vi "login.vi"() -> ()   [LabVIEW 2017]
panel:
  out "bandera 2":bool
  out "Usuarios dados de alta":string[][](array[string])
  out "Control":enum32{"LOGIN", "MENU 1", "MENU 2"}(tab)
  in  "ingresar  2":bool
  in  "Contraseña 2":string
  in  "Usuario 2":string
  in  "volver 3":bool
  in  "Agragar usuario 2":bool
  in  "Usuario  2":string
  in  "Contraseña 3":string
  out "Secion iniciada por: 2":string
  in  "eliminar 2":bool
  in  "Digite el usuario que desea eliminar 2":string
  in  "OK Button 2":bool
  in  "volver 4":bool
  out "bandera":bool
  out "Usuarios dados de alta":string[][](array[string])
  out "Control":enum32{"LOGIN", "MENU 1", "MENU 2"}(tab)
  in  "ingresar":bool
  in  "Contraseña":string
  in  "Usuario":string
  in  "volver":bool
  in  "Agragar usuario":bool
  in  "Usuario":string
  in  "Contraseña":string
  out "Secion iniciada por:":string
  in  "eliminar":bool
  in  "Digite el usuario que desea eliminar":string
  in  "OK Button":bool
  in  "volver 2":bool
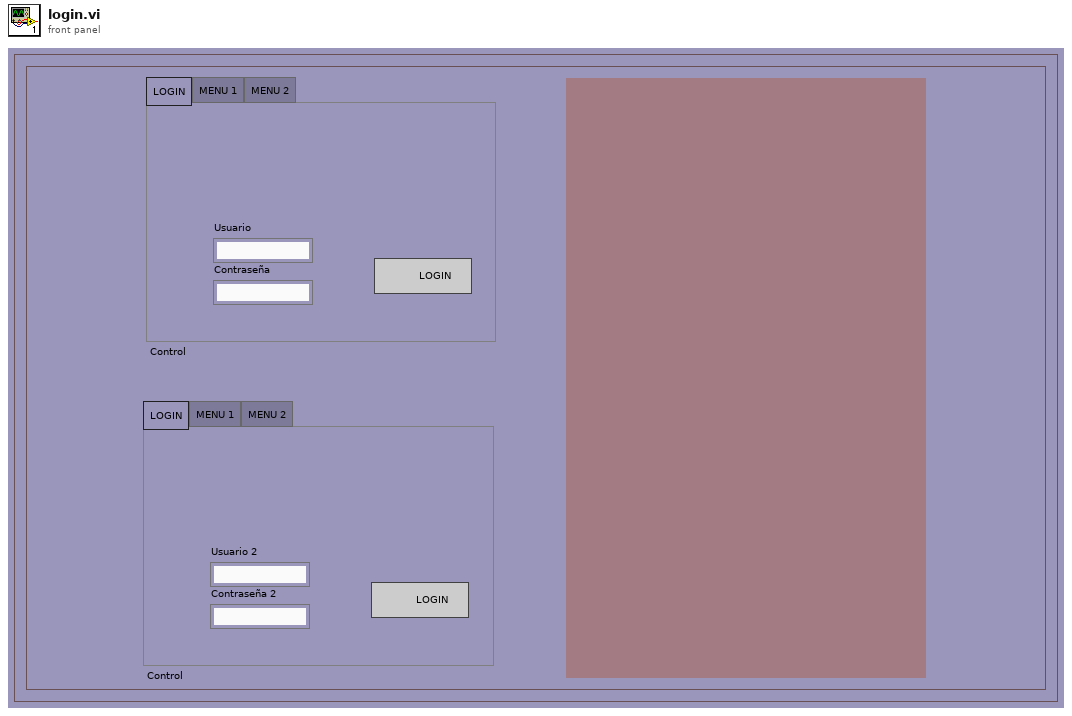
[diagram p1: front panel]
types:
  T1 = enum16{"open", "replace", "create", "open or create", "replace or create", "replace or create with confirmation"}
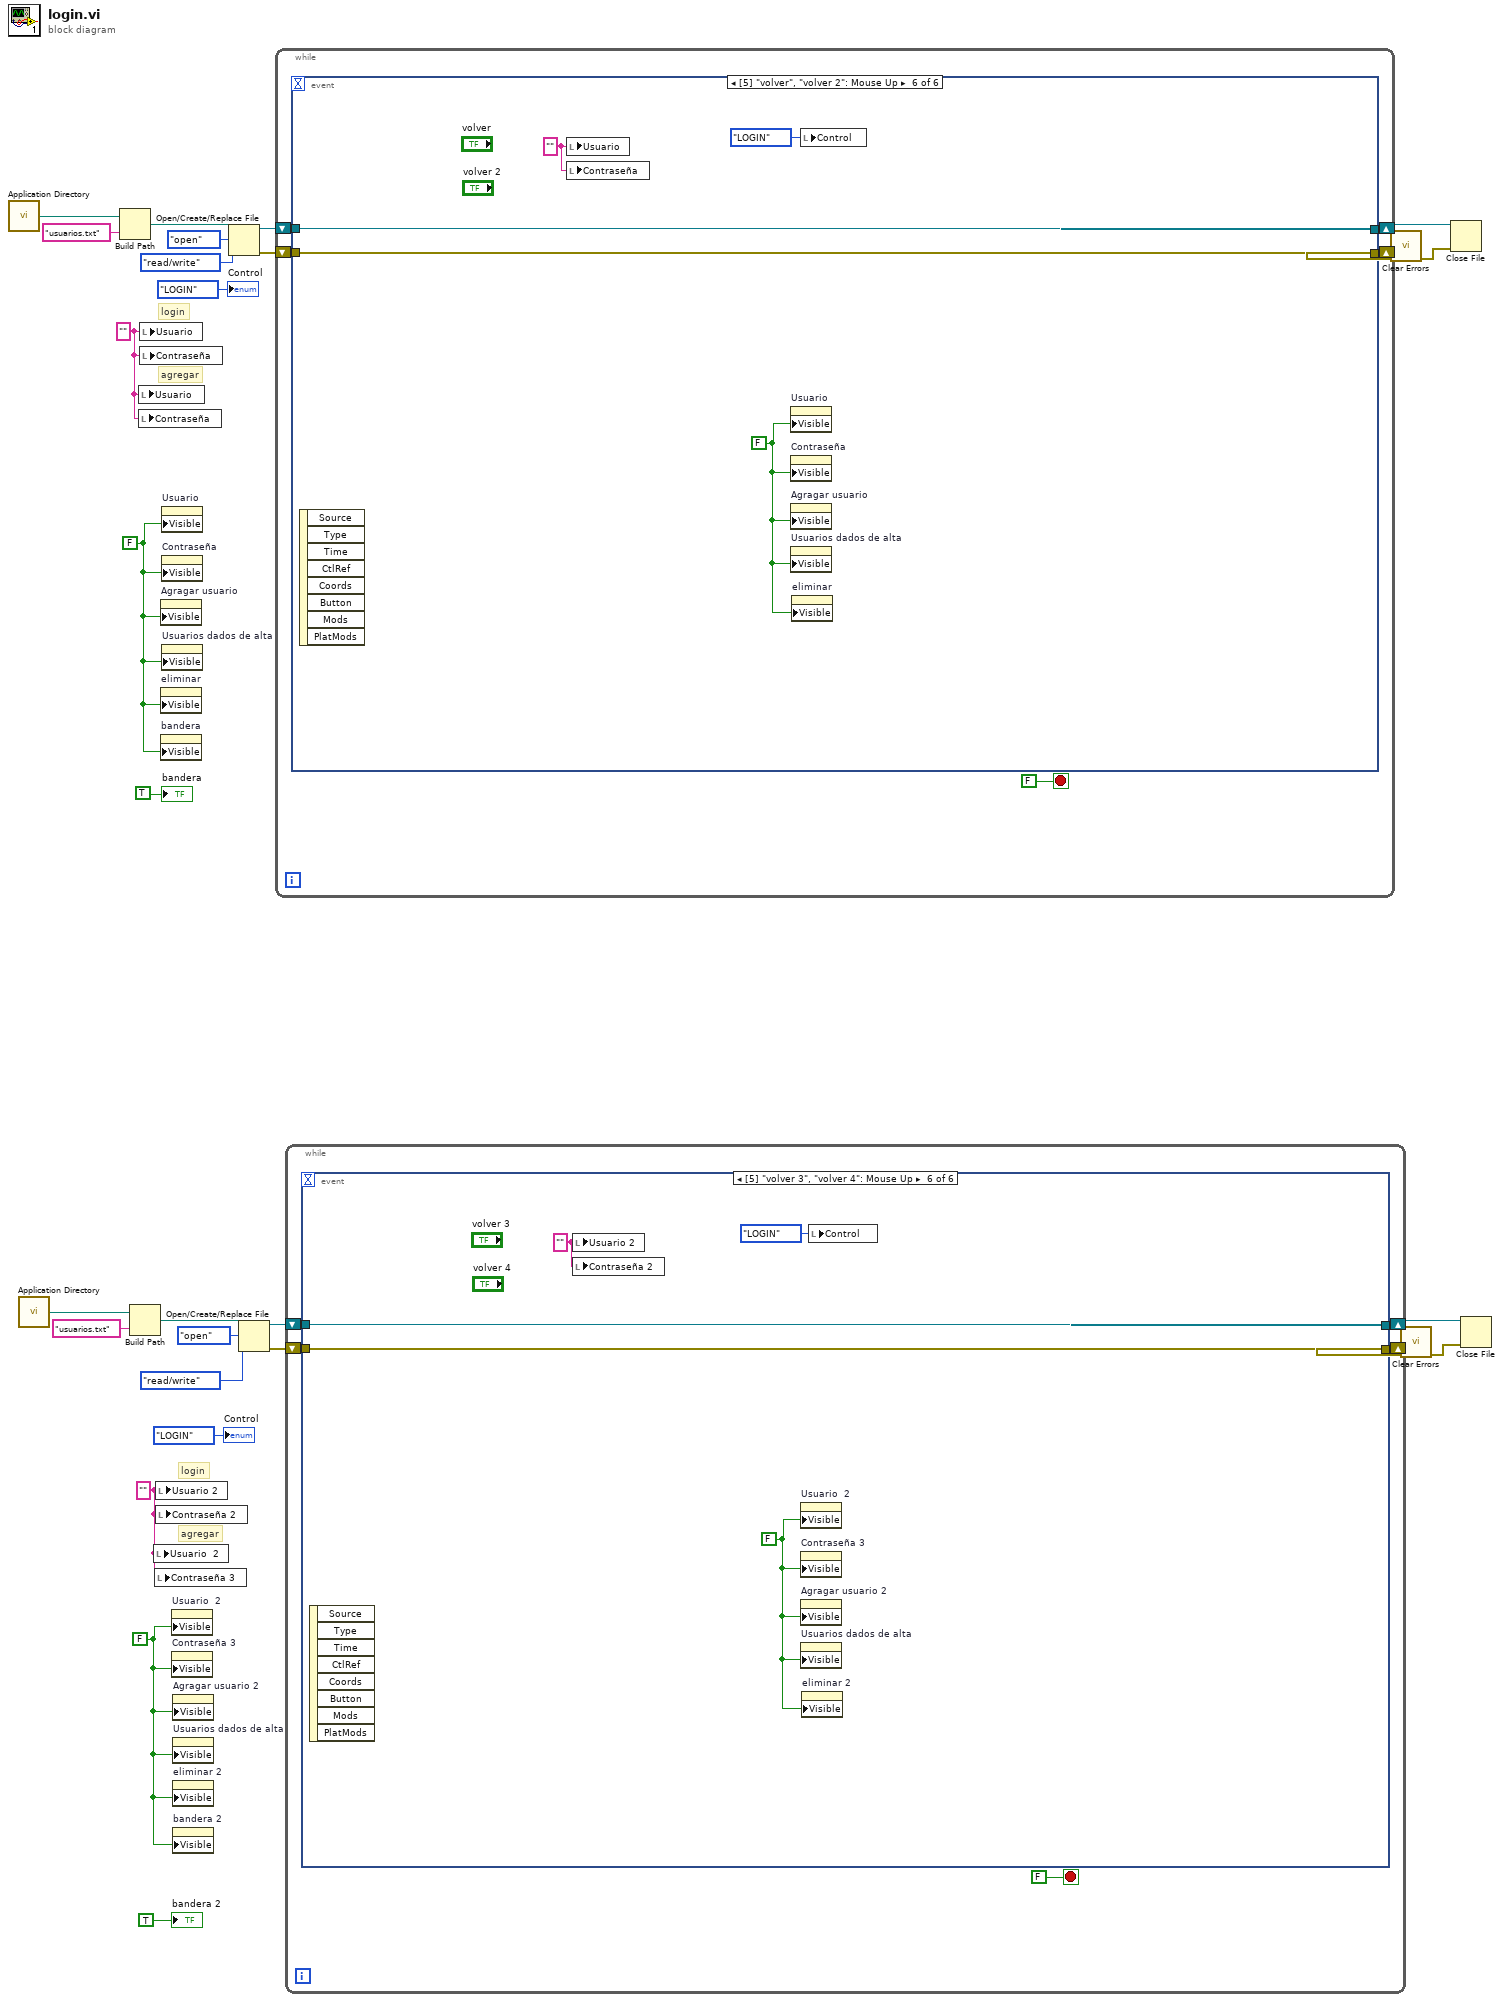
[diagram p0: block diagram]
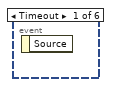
[diagram p2: hidden frame]
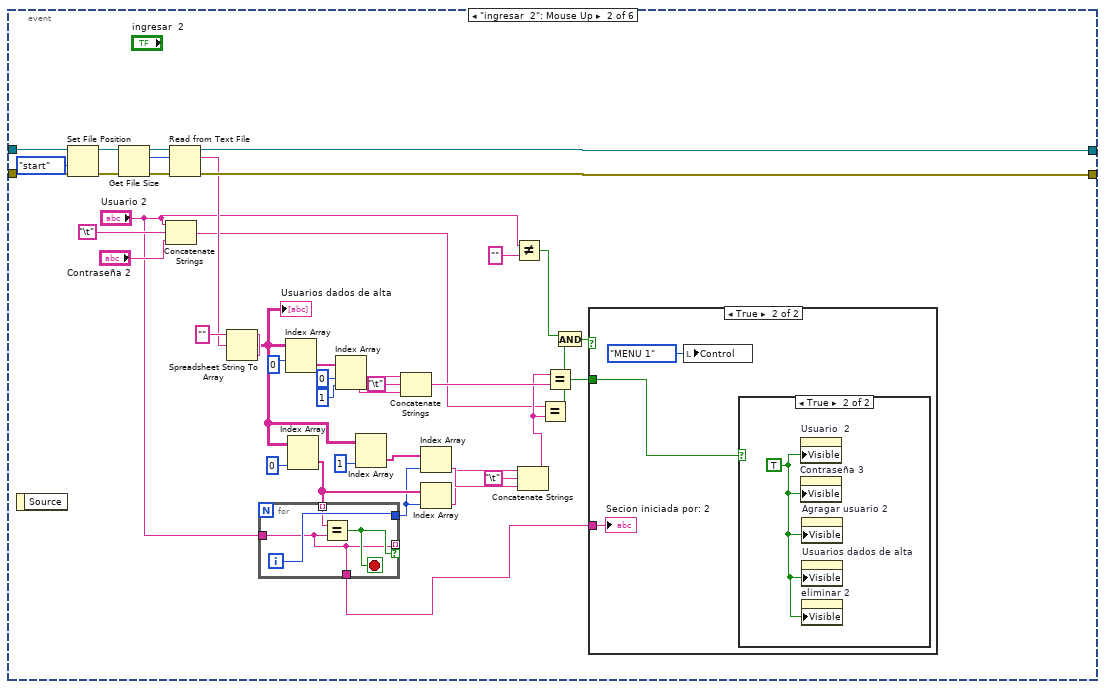
[diagram p3: hidden frame]
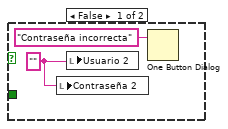
[diagram p4: hidden frame]
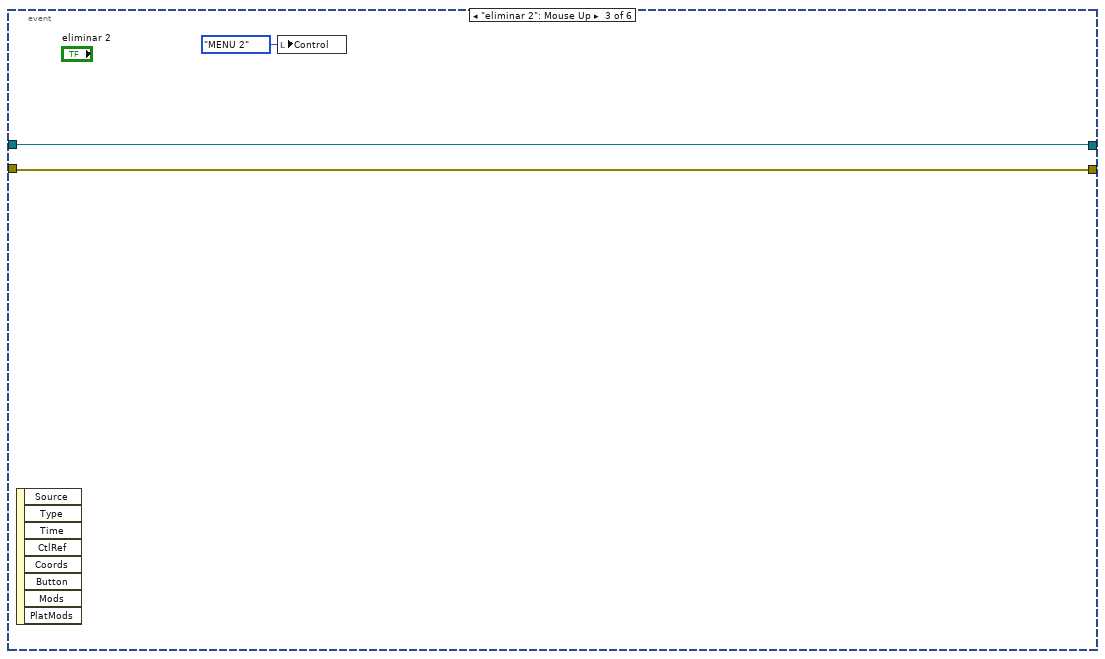
[diagram p6: hidden frame]
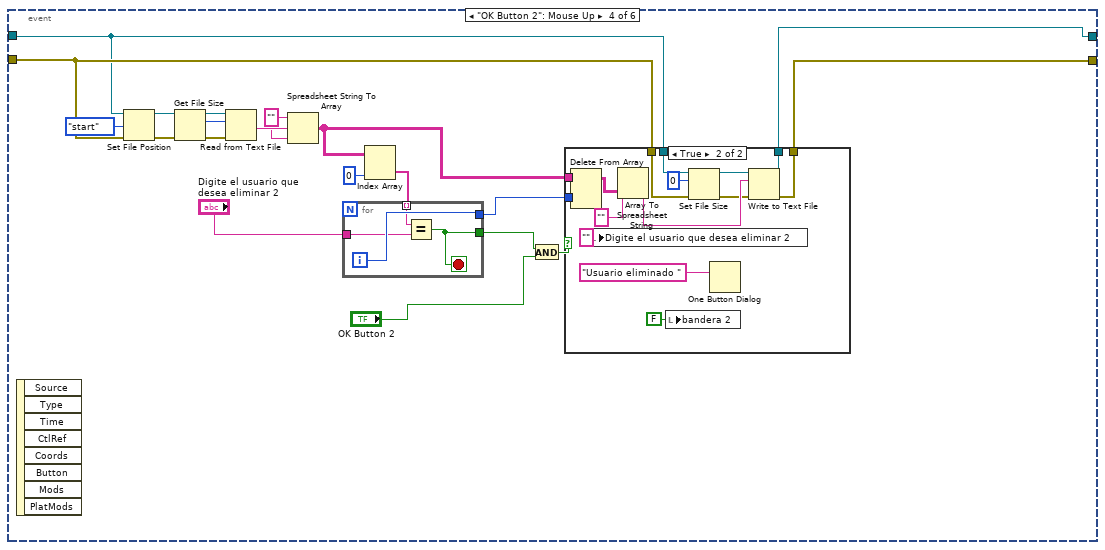
[diagram p7: hidden frame]
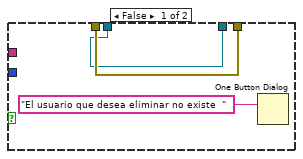
[diagram p8: hidden frame]
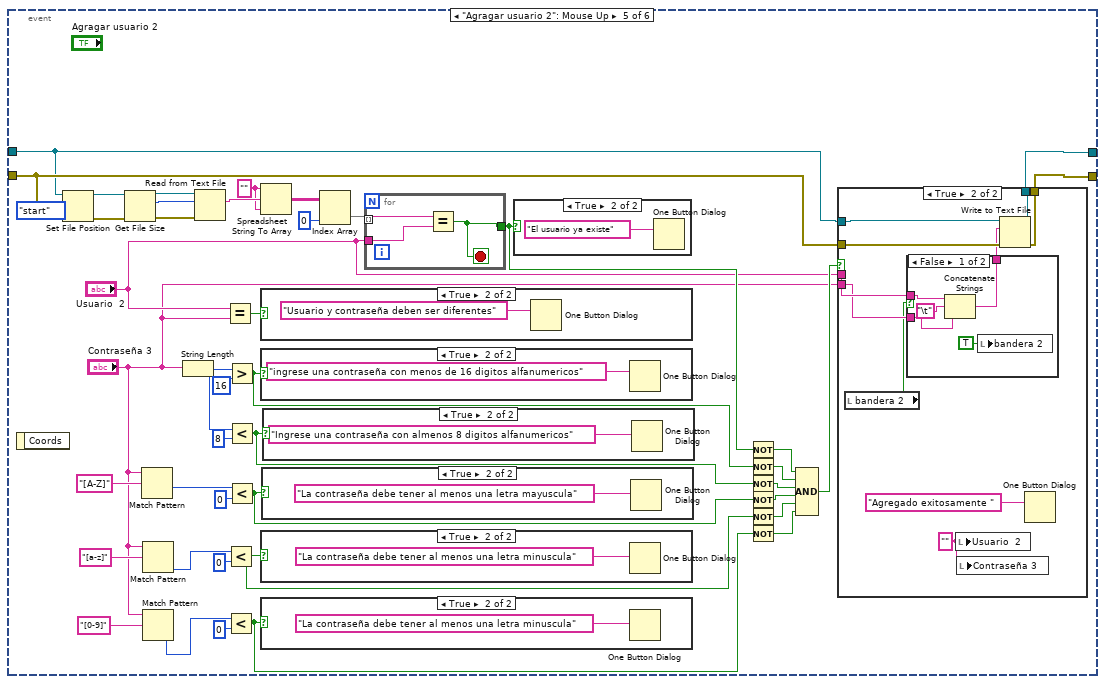
[diagram p9: hidden frame]
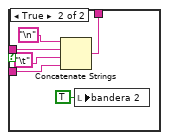
[diagram p11: hidden frame]
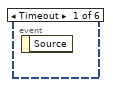
[diagram p19: hidden frame]
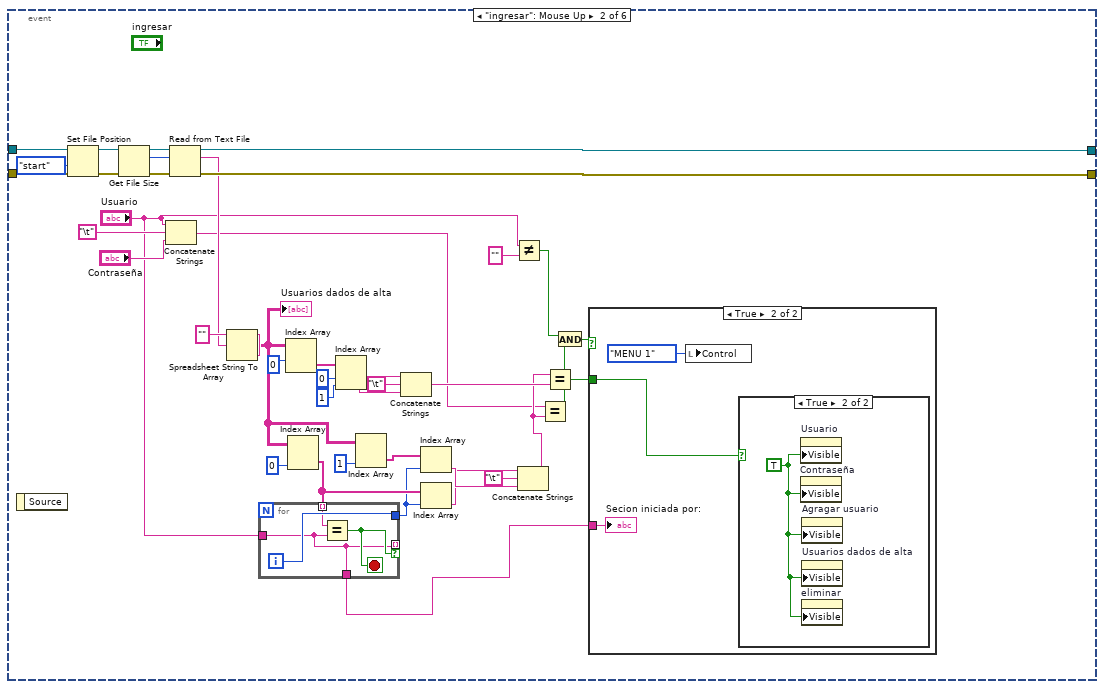
[diagram p20: hidden frame]
diagram:
  w2 = FALSE
  w4 = "" ("Usuario")
  w16 = FALSE
  w18 = "" ("Usuario")
  # "agregar"
  # "login"
  # "agregar"
  # "login"
  n1 = call <vilib>:"Application Directory.vi"() -> ("Application Directory"=w27:path)
  n2 = call <vilib>:"Application Directory.vi"() -> ("Application Directory"=w13:path)
  n3 = Build Path(base path=w27, name or relative path="usuarios.txt") -> (appended path=w26:path)
  n4 = Build Path(base path=w13, name or relative path="usuarios.txt") -> (appended path=w12:path)
  n5 = local write "Usuario"(w18) -> ()
  n6 = local write "Contraseña"(w18) -> ()
  n7 = local write "Usuario"(w18) -> ()
  n8 = local write "Contraseña"(w18) -> ()
  n9 = local write "Usuario  2"(w4) -> ()
  n10 = local write "Contraseña 3"(w4) -> ()
  n11 = local write "Usuario 2"(w4) -> ()
  n12 = local write "Contraseña 2"(w4) -> ()
  n13 = property on="Agragar usuario" class="Bool (strict)"("Visible"=w16) -> ()  [unwired: 2 in, 2 out]
  n14 = property on="eliminar" class="Bool (strict)"("Visible"=w16) -> ()  [unwired: 2 in, 2 out]
  n15 = property on="bandera" class="Bool (strict)"("Visible"=w16) -> ()  [unwired: 2 in, 2 out]
  n16 = property on="Usuario" class="Str"("Visible"=w16) -> ()  [unwired: 2 in, 2 out]
  n17 = property on="Contraseña" class="Str"("Visible"=w16) -> ()  [unwired: 2 in, 2 out]
  n18 = property on="Usuarios dados de alta" class="Arr (strict)"("Visible"=w16) -> ()  [unwired: 2 in, 2 out]
  n19 = property on="Usuario  2" class="Str"("Visible"=w2) -> ()  [unwired: 2 in, 2 out]
  n20 = property on="Contraseña 3" class="Str"("Visible"=w2) -> ()  [unwired: 2 in, 2 out]
  n21 = property on="Agragar usuario 2" class="Bool (strict)"("Visible"=w2) -> ()  [unwired: 2 in, 2 out]
  n22 = property on="Usuarios dados de alta" class="Arr (strict)"("Visible"=w2) -> ()  [unwired: 2 in, 2 out]
  n23 = property on="eliminar 2" class="Bool (strict)"("Visible"=w2) -> ()  [unwired: 2 in, 2 out]
  n24 = property on="bandera 2" class="Bool (strict)"("Visible"=w2) -> ()  [unwired: 2 in, 2 out]
  n25 = Open/Create/Replace File(file path (use dialog)=w26, operation (0:open)=T1."open", access (0:read/write)=enum16{"read/write", "read-only", "write-only"}."read/write") -> (refnum out=w23:refnum<file>, error out=w22:errorcluster)  [unwired: 3 in, 1 out]
  n26 = Open/Create/Replace File(file path (use dialog)=w12, operation (0:open)=T1."open", access (0:read/write)=enum16{"read/write", "read-only", "write-only"}."read/write") -> (refnum out=w9:refnum<file>, error out=w8:errorcluster)  [unwired: 3 in, 1 out]
  n27 = while {
    shift-right: [w29] -> w21
    shift-left: w22 -> [w31]
    shift-right: [w30] -> w19
    shift-left: w23 -> [w32]
    stop <- FALSE stop-if-true
    n28 = event shown="[5] \"volver\", \"volver 2\": Mouse Up" {
      selector: _ -> [_ _ _ _ _ _]
      dyn-events: _ -> [_ _ _ _ _ _]
      timeout: _ -> [_ _ _ _ _ _]
      tunnel: w32 -> [_ w73 w85 w89 w130 w209]
      tunnel: w31 -> [_ w72 w86 w90 w131 w208]
      tunnel: [_ w66 w85 w88 w133 w209] -> w30
      tunnel: [_ w65 w86 w87 w132 w208] -> w29
      event Timeout {
        n29 = event-data() -> ()  [unwired: 1 in, 1 out]
      }
      event "ingresar": Mouse Up {
        w62 = "" ("format string")
        n30 = event-data() -> ()  [unwired: 1 in, 1 out]
        n31 = Set File Position(refnum=w73, from (0:start)=enum16{"start", "end", "current"}."start", error in=w72) -> (refnum out=w71:refnum<file>, error out=w70:errorcluster)  [unwired: 1 in]
        n32 = Get File Size(file=w71, error in=w70) -> (refnum out=w69:refnum<file>, size (in bytes)=w67:i64, 0:w68:errorcluster)
        n33 = Concatenate Strings("Usuario", "\t", "Contraseña") -> (w39:string)
        n34 = Read from Text File(file (use dialog)=w69, count=w67, error in=w68) -> (refnum out=w66:refnum<file>, text=w53:string, error out=w65:errorcluster)  [unwired: 1 in, 1 out]
        n35 = Spreadsheet String To Array(format string=w62, spreadsheet string=w53, array type (2D Dbl)=w62) -> (array=w51:string[][])  [unwired: 1 in]
        "Usuarios dados de alta" <- w51
        n36 = Index Array(array=w51, index (row)=0) -> (element=w60:string[])  [unwired: 1 in]
        n37 = Index Array(array=w51, index (col)=0 ("disabled index (col)")) -> (element=w49:string[])  [unwired: 1 in]
        n38 = for {
          tunnel: "Usuario" -> [w75]
          tunnel: [w75] -> _ mode=indexing if=w77
          tunnel: [w76] -> w48
          tunnel: [w75] -> w43
          tunnel: w49 -> [w74] mode=indexing
          i -> [w76]
          stop <- w77 stop-if-true
          n39 = Equal?(x=w74, y=w75) -> (x = y?=w77:bool)
        }
        n40 = Index Array(array=w60, index #1=0 ("index"), index #2=1 ("index")) -> (element #1=w57:string, element #2=w55:string)
        n41 = Index Array(array=w51, index (col)=1 ("disabled index (col)")) -> (element=w47:string[])  [unwired: 1 in]
        n42 = Concatenate Strings(w57, "\t", w55) -> (w54:string)
        n43 = Index Array(array=w47, index=w48) -> (element=w45:string)
        n44 = Index Array(array=w49, index=w48) -> (element=w44:string)
        n45 = Not Equal?(x="Usuario", y="") -> (x != y?=w37:bool)
        n46 = Concatenate Strings(w44, "\t", w45) -> (w41:string)
        n47 = Equal?(x=w39, y=w41) -> (x = y?=w36:bool)
        n48 = Equal?(x=w41, y=w54) -> (x = y?=w42:bool)
        n49 = And(x=w37, y=w36) -> (x .and. y?=w35:bool)
        n50 = case shown="True" w35 {
          tunnel: w43 -> [_ w82]
          tunnel: w42 -> [_ w81]
          frame False {
            w78 = "" ("Usuario")
            n51 = local write "Contraseña"(w78) -> ()
            n52 = local write "Usuario"(w78) -> ()
            n53 = One Button Dialog(message="Contraseña incorrecta") -> ()  [unwired: 1 in, 1 out]
          }
          frame True {
            n54 = local write "Control"(enum32{"LOGIN", "MENU 1", "MENU 2"}."MENU 1" ("Control")) -> ()
            n55 = case shown="True" w81 {
              frame False {
              }
              frame True {
                w83 = TRUE
                n56 = property on="Usuario" class="Str"("Visible"=w83) -> ()  [unwired: 2 in, 2 out]
                n57 = property on="Contraseña" class="Str"("Visible"=w83) -> ()  [unwired: 2 in, 2 out]
                n58 = property on="Agragar usuario" class="Bool (strict)"("Visible"=w83) -> ()  [unwired: 2 in, 2 out]
                n59 = property on="Usuarios dados de alta" class="Arr (strict)"("Visible"=w83) -> ()  [unwired: 2 in, 2 out]
                n60 = property on="eliminar" class="Bool (strict)"("Visible"=w83) -> ()  [unwired: 2 in, 2 out]
              }
            }
            "Secion iniciada por:" <- w82
          }
        }
      }
      event "eliminar": Mouse Up {
        n61 = event-data() -> ()  [unwired: 1 in, 8 out]
        n62 = local write "Control"(enum32{"LOGIN", "MENU 1", "MENU 2"}."MENU 2" ("Control")) -> ()
      }
      event "OK Button": Mouse Up {
        w95 = "" ("format string")
        n63 = event-data() -> ()  [unwired: 1 in, 8 out]
        n64 = Set File Position(refnum=w89, from (0:start)=enum16{"start", "end", "current"}."start", error in=w90) -> (refnum out=w106:refnum<file>, error out=w105:errorcluster)  [unwired: 1 in]
        n65 = Get File Size(file=w106, error in=w105) -> (refnum out=w104:refnum<file>, size (in bytes)=w102:i64, 0:w103:errorcluster)
        n66 = Read from Text File(file (use dialog)=w104, count=w102, error in=w103) -> (text=w101:string)  [unwired: 1 in, 3 out]
        n67 = Spreadsheet String To Array(format string=w95, spreadsheet string=w101, array type (2D Dbl)=w95) -> (array=w92:string[][])  [unwired: 1 in]
        n68 = Index Array(array=w92, index (col)=0 ("disabled index (col)")) -> (element=w100:string[])  [unwired: 1 in]
        n69 = for {
          tunnel: "Digite el usuario que desea eliminar" -> [w127]
          tunnel: [w128] -> w91
          tunnel: w100 -> [w126] mode=indexing
          tunnel: [w125] -> w93
          i -> [w128]
          stop <- w125 stop-if-true
          n70 = Equal?(x=w126, y=w127) -> (x = y?=w125:bool)
        }
        n71 = And(x=w93, y="OK Button") -> (x .and. y?=w97:bool)
        n72 = case shown="True" w97 {
          tunnel: w92 -> [_ w122]
          tunnel: w91 -> [_ w121]
          tunnel: w90 -> [w109 w113]
          tunnel: w89 -> [w108 w112]
          tunnel: [w108 w120] -> w88
          tunnel: [w109 w119] -> w87
          frame False {
            n73 = One Button Dialog(message="El usuario que desea eliminar no existe  ") -> ()  [unwired: 1 in, 1 out]
          }
          frame True {
            n74 = Delete From Array(array=w122, index (row)=w121) -> (array with subset deleted=w118:string[][])  [unwired: 2 in, 1 out]
            n75 = local write "Digite el usuario que desea eliminar"("" ("Digite el usuario que desea eliminar")) -> ()
            n76 = Array To Spreadsheet String(array=w118, 3:"" ("format string")) -> (spreadsheet string=w116:string)  [unwired: 1 in]
            n77 = local write "bandera"(FALSE ("bandera")) -> ()
            n78 = Set File Size(4:w113, 6:i64 0 ("size (in bytes)"), 7:w112) -> (0:w114:errorcluster, 3:w115:refnum<file>)
            n79 = One Button Dialog(message="Usuario eliminado ") -> ()  [unwired: 1 in, 1 out]
            n80 = Write to Text File(file (use dialog)=w115, text=w116, error in=w114) -> (refnum out=w120:refnum<file>, error out=w119:errorcluster)  [unwired: 1 in, 1 out]
          }
        }
      }
      event "Agragar usuario": Mouse Up {
        w152 = "" ("format string")
        n81 = event-data() -> ()  [unwired: 1 in, 1 out]
        n82 = Set File Position(refnum=w130, from (0:start)=enum16{"start", "end", "current"}."start", error in=w131) -> (refnum out=w157:refnum<file>, error out=w158:errorcluster)  [unwired: 1 in]
        n83 = Get File Size(file=w157, error in=w158) -> (refnum out=w156:refnum<file>, size (in bytes)=w154:i64, 0:w155:errorcluster)
        n84 = Match Pattern(string="Contraseña", regular expression="[A-Z]") -> (offset past match=w167:i32)  [unwired: 1 in, 3 out]
        n85 = Match Pattern(string="Contraseña", regular expression="[a-z]") -> (offset past match=w163:i32)  [unwired: 1 in, 3 out]
        n86 = Match Pattern(string="Contraseña", regular expression="[0-9]") -> (offset past match=w160:i32)  [unwired: 1 in, 3 out]
        n87 = String Length(string="Contraseña") -> (length=w170:i32)
        n88 = Read from Text File(file (use dialog)=w156, count=w154, error in=w155) -> (text=w153:string)  [unwired: 1 in, 3 out]
        n89 = Equal?(x="Usuario", y="Contraseña") -> (x = y?=w159:bool)
        n90 = Less?(x=w163, y=0) -> (x < y?=w148:bool)
        n91 = Less?(x=w160, y=0) -> (x < y?=w144:bool)
        n92 = Greater?(x=w170, y=16) -> (0:w145:bool)
        n93 = Less?(x=w170, y=8) -> (x < y?=w146:bool)
        n94 = Less?(x=w167, y=0) -> (x < y?=w147:bool)
        n95 = Spreadsheet String To Array(format string=w152, spreadsheet string=w153, array type (2D Dbl)=w152) -> (array=w151:string[][])  [unwired: 1 in]
        n96 = case shown="True" w159 {
          frame False {
          }
          frame True {
            n97 = One Button Dialog(message="Usuario y contraseña deben ser diferentes") -> ()  [unwired: 1 in, 1 out]
          }
        }
        n98 = case shown="True" w145 {
          frame False {
          }
          frame True {
            n99 = One Button Dialog(message="ingrese una contraseña con menos de 16 digitos alfanumericos") -> ()  [unwired: 1 in, 1 out]
          }
        }
        n100 = case shown="True" w148 {
          frame False {
          }
          frame True {
            n101 = One Button Dialog(message="La contraseña debe tener al menos una letra minuscula") -> ()  [unwired: 1 in, 1 out]
          }
        }
        n102 = case shown="True" w144 {
          frame False {
          }
          frame True {
            n103 = One Button Dialog(message="La contraseña debe tener al menos una letra minuscula") -> ()  [unwired: 1 in, 1 out]
          }
        }
        n104 = case shown="True" w147 {
          frame False {
          }
          frame True {
            n105 = One Button Dialog(message="La contraseña debe tener al menos una letra mayuscula") -> ()  [unwired: 1 in, 1 out]
          }
        }
        n106 = case shown="True" w146 {
          frame False {
          }
          frame True {
            n107 = One Button Dialog(message="Ingrese una contraseña con almenos 8 digitos alfanumericos") -> ()  [unwired: 1 in, 1 out]
          }
        }
        n108 = Index Array(array=w151, index (col)=0 ("disabled index (col)")) -> (element=w149:string[])  [unwired: 1 in]
        n109 = for {
          tunnel: "Usuario" -> [w198]
          tunnel: w149 -> [w197] mode=indexing
          tunnel: [w196] -> w143
          stop <- w196 stop-if-true
          n110 = Equal?(x=w197, y=w198) -> (x = y?=w196:bool)
        }
        n111 = case shown="True" w143 {
          frame False {
          }
          frame True {
            n112 = One Button Dialog(message="El usuario ya existe") -> ()  [unwired: 1 in, 1 out]
          }
        }
        n113 = Not(x=w143) -> (.not. x?=w142:bool)
        n114 = Not(x=w145) -> (.not. x?=w138:bool)
        n115 = Not(x=w146) -> (.not. x?=w137:bool)
        n116 = Not(x=w147) -> (.not. x?=w139:bool)
        n117 = Not(x=w148) -> (.not. x?=w140:bool)
        n118 = Not(x=w144) -> (.not. x?=w141:bool)
        n119 = Compound Arithmetic op=AND(w142, w138, w137, w139, w140, w141) -> (w136:bool)
        n120 = case shown="True" w136 {
          tunnel: w130 -> [w173 w183]
          tunnel: w131 -> [w172 w182]
          tunnel: "Usuario" -> [_ w179]
          tunnel: "Contraseña" -> [_ w175]
          tunnel: [w173 w176] -> w133
          tunnel: [w172 w181] -> w132
          frame False {
          }
          frame True {
            w177 = "" ("Usuario")
            n121 = local read "bandera"() -> (w174:bool)
            n122 = case shown="False" w174 {
              tunnel: w179 -> [w188 w193]
              tunnel: [w186 w192] -> w178
              tunnel: w175 -> [w187 w190]
              frame False {
                n123 = Concatenate Strings(w188, "\t", w187) -> (w186:string)
                n124 = local write "bandera"(TRUE ("bandera")) -> ()
              }
              frame True {
                n125 = Concatenate Strings("\n", w193, "\t", w190) -> (w192:string)
                n126 = local write "bandera"(TRUE ("bandera")) -> ()
              }
            }
            n127 = local write "Usuario"(w177) -> ()
            n128 = local write "Contraseña"(w177) -> ()
            n129 = Write to Text File(file (use dialog)=w183, text=w178, error in=w182) -> (refnum out=w176:refnum<file>, error out=w181:errorcluster)  [unwired: 1 in, 1 out]
            n130 = One Button Dialog(message="Agregado exitosamente ") -> ()  [unwired: 1 in, 1 out]
          }
        }
      }
      event "volver", "volver 2": Mouse Up {
        w206 = FALSE
        w207 = "" ("Usuario")
        n131 = event-data() -> ()  [unwired: 1 in, 8 out]
        n132 = local write "Usuario"(w207) -> ()
        n133 = local write "Contraseña"(w207) -> ()
        n134 = property on="Usuario" class="Str"("Visible"=w206) -> ()  [unwired: 2 in, 2 out]
        n135 = property on="Contraseña" class="Str"("Visible"=w206) -> ()  [unwired: 2 in, 2 out]
        n136 = property on="Agragar usuario" class="Bool (strict)"("Visible"=w206) -> ()  [unwired: 2 in, 2 out]
        n137 = property on="Usuarios dados de alta" class="Arr (strict)"("Visible"=w206) -> ()  [unwired: 2 in, 2 out]
        n138 = property on="eliminar" class="Bool (strict)"("Visible"=w206) -> ()  [unwired: 2 in, 2 out]
        n139 = local write "Control"(enum32{"LOGIN", "MENU 1", "MENU 2"}."LOGIN" ("Control")) -> ()
      }
    }
  }
  n140 = while {
    shift-right: [w210] -> w7
    shift-left: w8 -> [w212]
    shift-right: [w211] -> w5
    shift-left: w9 -> [w213]
    stop <- FALSE stop-if-true
    n141 = event shown="[5] \"volver 3\", \"volver 4\": Mouse Up" {
      selector: _ -> [_ _ _ _ _ _]
      dyn-events: _ -> [_ _ _ _ _ _]
      timeout: _ -> [_ _ _ _ _ _]
      tunnel: w213 -> [_ w254 w266 w270 w311 w390]
      tunnel: w212 -> [_ w253 w267 w271 w312 w389]
      tunnel: [_ w247 w266 w269 w314 w390] -> w211
      tunnel: [_ w246 w267 w268 w313 w389] -> w210
      event Timeout {
        n142 = event-data() -> ()  [unwired: 1 in, 1 out]
      }
      event "ingresar  2": Mouse Up {
        w243 = "" ("format string")
        n143 = event-data() -> ()  [unwired: 1 in, 1 out]
        n144 = Set File Position(refnum=w254, from (0:start)=enum16{"start", "end", "current"}."start", error in=w253) -> (refnum out=w252:refnum<file>, error out=w251:errorcluster)  [unwired: 1 in]
        n145 = Get File Size(file=w252, error in=w251) -> (refnum out=w250:refnum<file>, size (in bytes)=w248:i64, 0:w249:errorcluster)
        n146 = Concatenate Strings("Usuario 2", "\t", "Contraseña 2") -> (w220:string)
        n147 = Read from Text File(file (use dialog)=w250, count=w248, error in=w249) -> (refnum out=w247:refnum<file>, text=w234:string, error out=w246:errorcluster)  [unwired: 1 in, 1 out]
        n148 = Spreadsheet String To Array(format string=w243, spreadsheet string=w234, array type (2D Dbl)=w243) -> (array=w232:string[][])  [unwired: 1 in]
        "Usuarios dados de alta" <- w232
        n149 = Index Array(array=w232, index (row)=0) -> (element=w241:string[])  [unwired: 1 in]
        n150 = Index Array(array=w232, index (col)=0 ("disabled index (col)")) -> (element=w230:string[])  [unwired: 1 in]
        n151 = for {
          tunnel: "Usuario 2" -> [w256]
          tunnel: [w256] -> _ mode=indexing if=w258
          tunnel: [w257] -> w229
          tunnel: [w256] -> w224
          tunnel: w230 -> [w255] mode=indexing
          i -> [w257]
          stop <- w258 stop-if-true
          n152 = Equal?(x=w255, y=w256) -> (x = y?=w258:bool)
        }
        n153 = Index Array(array=w241, index #1=0 ("index"), index #2=1 ("index")) -> (element #1=w238:string, element #2=w236:string)
        n154 = Index Array(array=w232, index (col)=1 ("disabled index (col)")) -> (element=w228:string[])  [unwired: 1 in]
        n155 = Concatenate Strings(w238, "\t", w236) -> (w235:string)
        n156 = Index Array(array=w228, index=w229) -> (element=w226:string)
        n157 = Index Array(array=w230, index=w229) -> (element=w225:string)
        n158 = Not Equal?(x="Usuario 2", y="") -> (x != y?=w218:bool)
        n159 = Concatenate Strings(w225, "\t", w226) -> (w222:string)
        n160 = Equal?(x=w220, y=w222) -> (x = y?=w217:bool)
        n161 = Equal?(x=w222, y=w235) -> (x = y?=w223:bool)
        n162 = And(x=w218, y=w217) -> (x .and. y?=w216:bool)
        n163 = case shown="True" w216 {
          tunnel: w224 -> [_ w263]
          tunnel: w223 -> [_ w262]
          frame False {
            w259 = "" ("Usuario")
            n164 = local write "Contraseña 2"(w259) -> ()
            n165 = local write "Usuario 2"(w259) -> ()
            n166 = One Button Dialog(message="Contraseña incorrecta") -> ()  [unwired: 1 in, 1 out]
          }
          frame True {
            n167 = local write "Control"(enum32{"LOGIN", "MENU 1", "MENU 2"}."MENU 1" ("Control")) -> ()
            n168 = case shown="True" w262 {
              frame False {
              }
              frame True {
                w264 = TRUE
                n169 = property on="Usuario  2" class="Str"("Visible"=w264) -> ()  [unwired: 2 in, 2 out]
                n170 = property on="Contraseña 3" class="Str"("Visible"=w264) -> ()  [unwired: 2 in, 2 out]
                n171 = property on="Agragar usuario 2" class="Bool (strict)"("Visible"=w264) -> ()  [unwired: 2 in, 2 out]
                n172 = property on="Usuarios dados de alta" class="Arr (strict)"("Visible"=w264) -> ()  [unwired: 2 in, 2 out]
                n173 = property on="eliminar 2" class="Bool (strict)"("Visible"=w264) -> ()  [unwired: 2 in, 2 out]
              }
            }
            "Secion iniciada por: 2" <- w263
          }
        }
      }
      event "eliminar 2": Mouse Up {
        n174 = event-data() -> ()  [unwired: 1 in, 8 out]
        n175 = local write "Control"(enum32{"LOGIN", "MENU 1", "MENU 2"}."MENU 2" ("Control")) -> ()
      }
      event "OK Button 2": Mouse Up {
        w276 = "" ("format string")
        n176 = event-data() -> ()  [unwired: 1 in, 8 out]
        n177 = Set File Position(refnum=w270, from (0:start)=enum16{"start", "end", "current"}."start", error in=w271) -> (refnum out=w287:refnum<file>, error out=w286:errorcluster)  [unwired: 1 in]
        n178 = Get File Size(file=w287, error in=w286) -> (refnum out=w285:refnum<file>, size (in bytes)=w283:i64, 0:w284:errorcluster)
        n179 = Read from Text File(file (use dialog)=w285, count=w283, error in=w284) -> (text=w282:string)  [unwired: 1 in, 3 out]
        n180 = Spreadsheet String To Array(format string=w276, spreadsheet string=w282, array type (2D Dbl)=w276) -> (array=w273:string[][])  [unwired: 1 in]
        n181 = Index Array(array=w273, index (col)=0 ("disabled index (col)")) -> (element=w281:string[])  [unwired: 1 in]
        n182 = for {
          tunnel: "Digite el usuario que desea eliminar 2" -> [w308]
          tunnel: [w309] -> w272
          tunnel: w281 -> [w307] mode=indexing
          tunnel: [w306] -> w274
          i -> [w309]
          stop <- w306 stop-if-true
          n183 = Equal?(x=w307, y=w308) -> (x = y?=w306:bool)
        }
        n184 = And(x=w274, y="OK Button 2") -> (x .and. y?=w278:bool)
        n185 = case shown="True" w278 {
          tunnel: w273 -> [_ w303]
          tunnel: w272 -> [_ w302]
          tunnel: w271 -> [w290 w294]
          tunnel: w270 -> [w289 w293]
          tunnel: [w289 w301] -> w269
          tunnel: [w290 w300] -> w268
          frame False {
            n186 = One Button Dialog(message="El usuario que desea eliminar no existe  ") -> ()  [unwired: 1 in, 1 out]
          }
          frame True {
            n187 = Delete From Array(array=w303, index (row)=w302) -> (array with subset deleted=w299:string[][])  [unwired: 2 in, 1 out]
            n188 = local write "Digite el usuario que desea eliminar 2"("" ("Digite el usuario que desea eliminar")) -> ()
            n189 = Array To Spreadsheet String(array=w299, 3:"" ("format string")) -> (spreadsheet string=w297:string)  [unwired: 1 in]
            n190 = local write "bandera 2"(FALSE ("bandera")) -> ()
            n191 = Set File Size(4:w294, 6:i64 0 ("size (in bytes)"), 7:w293) -> (0:w295:errorcluster, 3:w296:refnum<file>)
            n192 = One Button Dialog(message="Usuario eliminado ") -> ()  [unwired: 1 in, 1 out]
            n193 = Write to Text File(file (use dialog)=w296, text=w297, error in=w295) -> (refnum out=w301:refnum<file>, error out=w300:errorcluster)  [unwired: 1 in, 1 out]
          }
        }
      }
      event "Agragar usuario 2": Mouse Up {
        w333 = "" ("format string")
        n194 = event-data() -> ()  [unwired: 1 in, 1 out]
        n195 = Set File Position(refnum=w311, from (0:start)=enum16{"start", "end", "current"}."start", error in=w312) -> (refnum out=w338:refnum<file>, error out=w339:errorcluster)  [unwired: 1 in]
        n196 = Get File Size(file=w338, error in=w339) -> (refnum out=w337:refnum<file>, size (in bytes)=w335:i64, 0:w336:errorcluster)
        n197 = Match Pattern(string="Contraseña 3", regular expression="[A-Z]") -> (offset past match=w348:i32)  [unwired: 1 in, 3 out]
        n198 = Match Pattern(string="Contraseña 3", regular expression="[a-z]") -> (offset past match=w344:i32)  [unwired: 1 in, 3 out]
        n199 = Match Pattern(string="Contraseña 3", regular expression="[0-9]") -> (offset past match=w341:i32)  [unwired: 1 in, 3 out]
        n200 = String Length(string="Contraseña 3") -> (length=w351:i32)
        n201 = Read from Text File(file (use dialog)=w337, count=w335, error in=w336) -> (text=w334:string)  [unwired: 1 in, 3 out]
        n202 = Equal?(x="Usuario  2", y="Contraseña 3") -> (x = y?=w340:bool)
        n203 = Less?(x=w344, y=0) -> (x < y?=w329:bool)
        n204 = Less?(x=w341, y=0) -> (x < y?=w325:bool)
        n205 = Greater?(x=w351, y=16) -> (0:w326:bool)
        n206 = Less?(x=w351, y=8) -> (x < y?=w327:bool)
        n207 = Less?(x=w348, y=0) -> (x < y?=w328:bool)
        n208 = Spreadsheet String To Array(format string=w333, spreadsheet string=w334, array type (2D Dbl)=w333) -> (array=w332:string[][])  [unwired: 1 in]
        n209 = case shown="True" w340 {
          frame False {
          }
          frame True {
            n210 = One Button Dialog(message="Usuario y contraseña deben ser diferentes") -> ()  [unwired: 1 in, 1 out]
          }
        }
        n211 = case shown="True" w326 {
          frame False {
          }
          frame True {
            n212 = One Button Dialog(message="ingrese una contraseña con menos de 16 digitos alfanumericos") -> ()  [unwired: 1 in, 1 out]
          }
        }
        n213 = case shown="True" w329 {
          frame False {
          }
          frame True {
            n214 = One Button Dialog(message="La contraseña debe tener al menos una letra minuscula") -> ()  [unwired: 1 in, 1 out]
          }
        }
        n215 = case shown="True" w325 {
          frame False {
          }
          frame True {
            n216 = One Button Dialog(message="La contraseña debe tener al menos una letra minuscula") -> ()  [unwired: 1 in, 1 out]
          }
        }
        n217 = case shown="True" w328 {
          frame False {
          }
          frame True {
            n218 = One Button Dialog(message="La contraseña debe tener al menos una letra mayuscula") -> ()  [unwired: 1 in, 1 out]
          }
        }
        n219 = case shown="True" w327 {
          frame False {
          }
          frame True {
            n220 = One Button Dialog(message="Ingrese una contraseña con almenos 8 digitos alfanumericos") -> ()  [unwired: 1 in, 1 out]
          }
        }
        n221 = Index Array(array=w332, index (col)=0 ("disabled index (col)")) -> (element=w330:string[])  [unwired: 1 in]
        n222 = for {
          tunnel: "Usuario  2" -> [w379]
          tunnel: w330 -> [w378] mode=indexing
          tunnel: [w377] -> w324
          stop <- w377 stop-if-true
          n223 = Equal?(x=w378, y=w379) -> (x = y?=w377:bool)
        }
        n224 = case shown="True" w324 {
          frame False {
          }
          frame True {
            n225 = One Button Dialog(message="El usuario ya existe") -> ()  [unwired: 1 in, 1 out]
          }
        }
        n226 = Not(x=w324) -> (.not. x?=w323:bool)
        n227 = Not(x=w326) -> (.not. x?=w319:bool)
        n228 = Not(x=w327) -> (.not. x?=w318:bool)
        n229 = Not(x=w328) -> (.not. x?=w320:bool)
        n230 = Not(x=w329) -> (.not. x?=w321:bool)
        n231 = Not(x=w325) -> (.not. x?=w322:bool)
        n232 = Compound Arithmetic op=AND(w323, w319, w318, w320, w321, w322) -> (w317:bool)
        n233 = case shown="True" w317 {
          tunnel: w311 -> [w354 w364]
          tunnel: w312 -> [w353 w363]
          tunnel: "Usuario  2" -> [_ w360]
          tunnel: "Contraseña 3" -> [_ w356]
          tunnel: [w354 w357] -> w314
          tunnel: [w353 w362] -> w313
          frame False {
          }
          frame True {
            w358 = "" ("Usuario")
            n234 = local read "bandera 2"() -> (w355:bool)
            n235 = case shown="False" w355 {
              tunnel: w360 -> [w369 w374]
              tunnel: [w367 w373] -> w359
              tunnel: w356 -> [w368 w371]
              frame False {
                n236 = Concatenate Strings(w369, "\t", w368) -> (w367:string)
                n237 = local write "bandera 2"(TRUE ("bandera")) -> ()
              }
              frame True {
                n238 = Concatenate Strings("\n", w374, "\t", w371) -> (w373:string)
                n239 = local write "bandera 2"(TRUE ("bandera")) -> ()
              }
            }
            n240 = local write "Usuario  2"(w358) -> ()
            n241 = local write "Contraseña 3"(w358) -> ()
            n242 = Write to Text File(file (use dialog)=w364, text=w359, error in=w363) -> (refnum out=w357:refnum<file>, error out=w362:errorcluster)  [unwired: 1 in, 1 out]
            n243 = One Button Dialog(message="Agregado exitosamente ") -> ()  [unwired: 1 in, 1 out]
          }
        }
      }
      event "volver 3", "volver 4": Mouse Up {
        w387 = FALSE
        w388 = "" ("Usuario")
        n244 = event-data() -> ()  [unwired: 1 in, 8 out]
        n245 = local write "Usuario 2"(w388) -> ()
        n246 = local write "Contraseña 2"(w388) -> ()
        n247 = property on="Usuario  2" class="Str"("Visible"=w387) -> ()  [unwired: 2 in, 2 out]
        n248 = property on="Contraseña 3" class="Str"("Visible"=w387) -> ()  [unwired: 2 in, 2 out]
        n249 = property on="Agragar usuario 2" class="Bool (strict)"("Visible"=w387) -> ()  [unwired: 2 in, 2 out]
        n250 = property on="Usuarios dados de alta" class="Arr (strict)"("Visible"=w387) -> ()  [unwired: 2 in, 2 out]
        n251 = property on="eliminar 2" class="Bool (strict)"("Visible"=w387) -> ()  [unwired: 2 in, 2 out]
        n252 = local write "Control"(enum32{"LOGIN", "MENU 1", "MENU 2"}."LOGIN" ("Control")) -> ()
      }
    }
  }
  n253 = call <vilib>:"Clear Errors.vi"("error in (no error)"=w21) -> ("error out"=w20:errorcluster)  [unwired: 5 in, 1 out]
  n254 = call <vilib>:"Clear Errors.vi"("error in (no error)"=w7) -> ("error out"=w6:errorcluster)  [unwired: 5 in, 1 out]
  n255 = Close File(refnum=w19, error in=w20) -> ()  [unwired: 2 out]
  n256 = Close File(refnum=w5, error in=w6) -> ()  [unwired: 2 out]
  "Control" <- enum32{"LOGIN", "MENU 1", "MENU 2"}."LOGIN" ("Control")
  "bandera" <- TRUE ("bandera")
  "Control" <- enum32{"LOGIN", "MENU 1", "MENU 2"}."LOGIN" ("Control")
  "bandera 2" <- TRUE ("bandera")
